vi "LIA7230Monitor.vi"(0 "Lock-in Reference":u16(ring) items=["Lock-in 1", "Lock-in 2", "Lock-in 3"]) -> ()   [LabVIEW 2019]
uses:
  Utility/Monitor Communication/LIA7230/LIA7230-cluster.ctl
  Utility/Monitor Communication/LIA7230/Settings_cluster.ctl
  Instrument_Setup.vi
  Global/Global Variables/Data_Display_global.vi
panel:
  out "LIA7230-Settings":T1={"Interface"=1, "Port"=0, "Serial Number"="08199244", "IP Address"="192.168.11.6", "Line Frequency\nRejection Filter"=0, "Input Mode"=1, "Input Conn. Shells"=TRUE, "Line Frequency"=FALSE, "Auto AC Gain"=FALSE, "AC Gain"=0, "Input Device"=FALSE, "Range"=26, " Auto Sensitivity "=FALSE, "Auto Measure"=FALSE, "Range 2"=25, " Auto Sensitivity  2"=FALSE, "Slope"=1, "Synchronous TC"=FALSE, "Time Constant"=12, "Slope 2"=1, "Time Constant 2"=12, "Oscillator Amp (V rms)"=0.5, "Oscillator Freq (Hz)"=150000.0, "Reference I/P"=0, "Ref Harm 1"=1, "Ref Harm2"=2, "Virtual Ref.\nMode"=FALSE, "Dual Harmonic/Reference Mode"=FALSE, "Reference Mode"=FALSE, "TRIG OUT\n= Ref Mon"=FALSE, " Auto Phase "=FALSE, "Reference Phase 1"=0.0, "+90 degrees 1"=FALSE, " Auto Phase 2 "=FALSE, "Reference 2 Phase"=0.0, "+90 degrees2"=FALSE, "Auxiliary I/O"=FALSE, "Configuration"=FALSE, "Curve Buffer"=FALSE, "Offsets"=FALSE, "X Channel Offset (%)"=-6.7055225e-06, "X Channel Offset"=FALSE, "Y Channel Offset (%)"=-6.705522537231445e-06, "Y Channel Offset"=FALSE, " Auto Offset"=FALSE, "X Channel Offset (%) 2"=-6.7055225e-06, "X Channel Offset 2"=FALSE, "Y Channel Offset (%) 2"=-6.705522537231445e-06, "Y Channel Offset 2"=FALSE, " Auto Offset 2"=FALSE, "Display Type channel 1"=5, "Display Type channel 2"=5, "Display Type channel 3"=5, "Display Type channel 4"=5, "Osc Sweeps"=FALSE, "Define Equation1"=FALSE, "Coupling"=FALSE} {"Display Type channel 4" items=["X %", "Y %", "X Calibrated", "Y Calibrated", "Mag %", "Mag Calibrated", "Phase Degrees", "Ratio", "Log Ratio", "ADC 1", "ADC 2", "ADC 3", "ADC 4", "Noise %", "Noise Calibrated", "Ref Frequency", "Equation 1", "Equation 2", "X2 %", "Y2 %", "X2 Calibrated", "Y2 Calibrated", "Mag2 %", "Mag2 Calibrated", "Phase2 Degrees"]; "Display Type channel 3" items=["X %", "Y %", "X Calibrated", "Y Calibrated", "Mag %", "Mag Calibrated", "Phase Degrees", "Ratio", "Log Ratio", "ADC 1", "ADC 2", "ADC 3", "ADC 4", "Noise %", "Noise Calibrated", "Ref Frequency", "Equation 1", "Equation 2", "X2 %", "Y2 %", "X2 Calibrated", "Y2 Calibrated", "Mag2 %", "Mag2 Calibrated", "Phase2 Degrees"]; "Display Type channel 2" items=["X %", "Y %", "X Calibrated", "Y Calibrated", "Mag %", "Mag Calibrated", "Phase Degrees", "Ratio", "Log Ratio", "ADC 1", "ADC 2", "ADC 3", "ADC 4", "Noise %", "Noise Calibrated", "Ref Frequency", "Equation 1", "Equation 2", "X2 %", "Y2 %", "Mag2 %", "Mag2 Calibrated", "Phase2 Degrees"]; "Display Type channel 1" items=["X %", "Y %", "X Calibrated", "Y Calibrated", "Mag %", "Mag Calibrated", "Phase Degrees", "Ratio", "Log Ratio", "ADC 1", "ADC 2", "ADC 3", "ADC 4", "Noise %", "Noise Calibrated", "Ref Frequency", "Equation 1", "Equation 2", "X2 %", "Y2 %", "Mag2 %", "Mag2 Calibrated", "Phase2 Degrees"]; "Y Channel Offset (%) 2" format="%.2f"; "X Channel Offset (%) 2" min=-300 max=300 step=0.01 format="%.2f"; "Y Channel Offset (%)" format="%.2f"; "X Channel Offset (%)" min=-300 max=300 step=0.01 format="%.2f"; "Reference 2 Phase" min=-200.0 max=200.0 step=0.01 scale=-180.0..180.0 scale format="%.1f"; "Reference Phase 1" min=-200.0 max=200.0 step=0.01 scale=-180.0..180.0 scale format="%.1f"; "Ref Harm2" min=1 max=127 step=1; "Ref Harm 1" min=1 max=127 step=1; "Reference I/P" items=["Internal", "External TTL (Rear Panel)", "External (Front Panel)"]; "Oscillator Freq (Hz)" min=0.5 max=150000.0 step=0.001 format="%.3f"; "Oscillator Amp (V rms)" min=0.0 max=5.0 step=0.0001 format="%.3f"; "Time Constant 2" items=["10µs", "20µs", "50µs", "100µs", "200µs", "500µs", "1ms", "2ms", "5ms", "10ms", "20ms", "50ms", "100ms", "200ms", "500ms", "1s", "2s", "5s", "10s", "20s", "50s", "100s", "200s", "500s", "1ks", "2ks", "5ks", "10ks", "20ks", "50ks", "100ks"]; "Slope 2" items=["6db/octave", "12dB/octave", "18dB/octave", "24dB/octave"]; "Time Constant" items=["10µs", "20µs", "50µs", "100µs", "200µs", "500µs", "1ms", "2ms", "5ms", "10ms", "20ms", "50ms", "100ms", "200ms", "500ms", "1s", "2s", "5s", "10s", "20s", "50s", "100s", "200s", "500s", "1ks", "2ks", "5ks", "10ks", "20ks", "50ks", "100ks"]; "Slope" items=["6db/octave", "12dB/octave", "18dB/octave", "24dB/octave"]; "Range 2" items=["N/A", "2nV", "5nV", "10nV", "20nV", "50nV", "100nV", "200nV", "500nV", "1µV", "2µV", "5µV", "10µV", "20µV", "50µV", "100µV", "200µV", "500µV", "1mV", "2mV", "5mV", "10mV", "20mV", "50mV", "100mV", "200mV", "500mV", "1V"]; "Range" items=["N/A", "2nV", "5nV", "10nV", "20nV", "50nV", "100nV", "200nV", "500nV", "1µV", "2µV", "5µV", "10µV", "20µV", "50µV", "100µV", "200µV", "500µV", "1mV", "2mV", "5mV", "10mV", "20mV", "50mV", "100mV", "200mV", "500mV", "1V"]; "AC Gain" items=["0dB", "6dB", "12dB", "18dB", "24dB", "30dB", "36dB", "42dB", "48dB", "54dB", "60dB", "66dB", "78dB", "84dB", "90dB"]; "Input Mode" items=["Inputs Grounded (test)", "A (Single-Ended Voltage)", "-B (Inverting Single Ended Voltage)", "A-B (Differential Voltage)", "AUX Input - Main Console", "B Current input - Wide Bandwidth", "B Current input - Low Noise"]; "Line Frequency\nRejection Filter" items=["OFF", "F", "2F", "F & 2F"]; "Port" items=["COM 1", "COM 2", "COM 3", "COM 4", "COM 5", "COM 6", "COM 7", "COM 8", "COM 9", "COM 10"]; "Interface" items=["RS232", "USB", "Ethernet"]}
  out "Sensitivity Range dual mode":i16(ring)=15 items=["2 nV", "5 nV", "10 nV", "20 nV", "50 nV", "100 nV", "200 nV", "500 nV", "1 µV", "2 µV", "5 µV", "10 µV", "20 µV", "50 µV", "100 µV", "200 µV", "500 µV", "1 mV", "2 mV", "5 mV", "10 mV", "20 mV", "50 mV", "100 mV", "200 mV", "500 mV", "1 V", ""]
  out "LIA7230-Cluser":T2={"Lockin 1"=[], "X1-Display"=0.0, "X1 Percent"=0.0, "Y1-Display"=0.0, "X1 Percent 2"=0.0, "Unit X1"="nV", "Unit X2"="nV", "X1 Overload"=FALSE, "Y1 Overload"=FALSE, "Sensitivity Setpoint"=26, "X1"=0.0, "Y1"=0.0, "Channel 3"=0.0, "Channel 4"=0.0, "Channel 4 Percent"=0.0, "Channel 3 Percent "=0.0, "Unit Channel 3"="nV", "Unit Channel 4"="nV", "Overload channel 3"=FALSE, "Overload channel 4"=FALSE, "Offsets (ON)"=FALSE, "Sensitivity Setpoint 2"=26} {"Sensitivity Setpoint 2" items=["2 nV", "5 nV", "10 nV", "20 nV", "50 nV", "100 nV", "200 nV", "500 nV", "1 µV", "2 µV", "5 µV", "10 µV", "20 µV", "50 µV", "100 µV", "200 µV", "500 µV", "1 mV", "2 mV", "5 mV", "10 mV", "20 mV", "50 mV", "100 mV", "200 mV", "500 mV", "1 V", ""]; "Channel 3 Percent" scale=0.0..100.0; "Channel 4 Percent" scale=0.0..100.0; "Sensitivity Setpoint" items=["2 nV", "5 nV", "10 nV", "20 nV", "50 nV", "100 nV", "200 nV", "500 nV", "1 µV", "2 µV", "5 µV", "10 µV", "20 µV", "50 µV", "100 µV", "200 µV", "500 µV", "1 mV", "2 mV", "5 mV", "10 mV", "20 mV", "50 mV", "100 mV", "200 mV", "500 mV", "1 V", ""]; "X1 Percent 2" scale=0.0..100.0; "X1 Percent" scale=0.0..100.0; "X1-Display" format="%#4_5f"}
  out "Sensitivity Range single mode":i16(ring)=15 items=["2 nV", "5 nV", "10 nV", "20 nV", "50 nV", "100 nV", "200 nV", "500 nV", "1 µV", "2 µV", "5 µV", "10 µV", "20 µV", "50 µV", "100 µV", "200 µV", "500 µV", "1 mV", "2 mV", "5 mV", "10 mV", "20 mV", "50 mV", "100 mV", "200 mV", "500 mV", "1 V", ""]
  in  "Stopp":bool
  # "USB Interface"
  # "Ethernet Interface"
  # "Oscillator"
  # "Output Channels -Offset"
  # "Reference Control"
  # "Dual Reference/\nDual Harmonic"
  # "Single Reference/\nSingle Harmonic"
  # "Dual"
  # "Input Configuration"
  # "Output Channels TC & Slope"
  # "Single"
  # "On"
  # "On"
  # "Single mode"
  # "Dual mode"
  # "Off"
  # "Off"
  # "DC"
  # "Dual Ref. Mode"
  # "AC"
  # "Dual Harm. Mode"
  # "On"
  # "On"
  # "Off"
  # "Off"
  # "On"
  # "Float"
  # "On"
  # "On"
  # "Off"
  # "Ground"
  # "Off"
  # "Off"
  # "FET"
  # "Sensitivity"
  # "50 Hz"
  # "On"
  # "Dual mode"
  # "Single mode"
  # "Bipolar"
  # "60 Hz"
  # "Off"
  # "Degrees"
  # "Degrees"
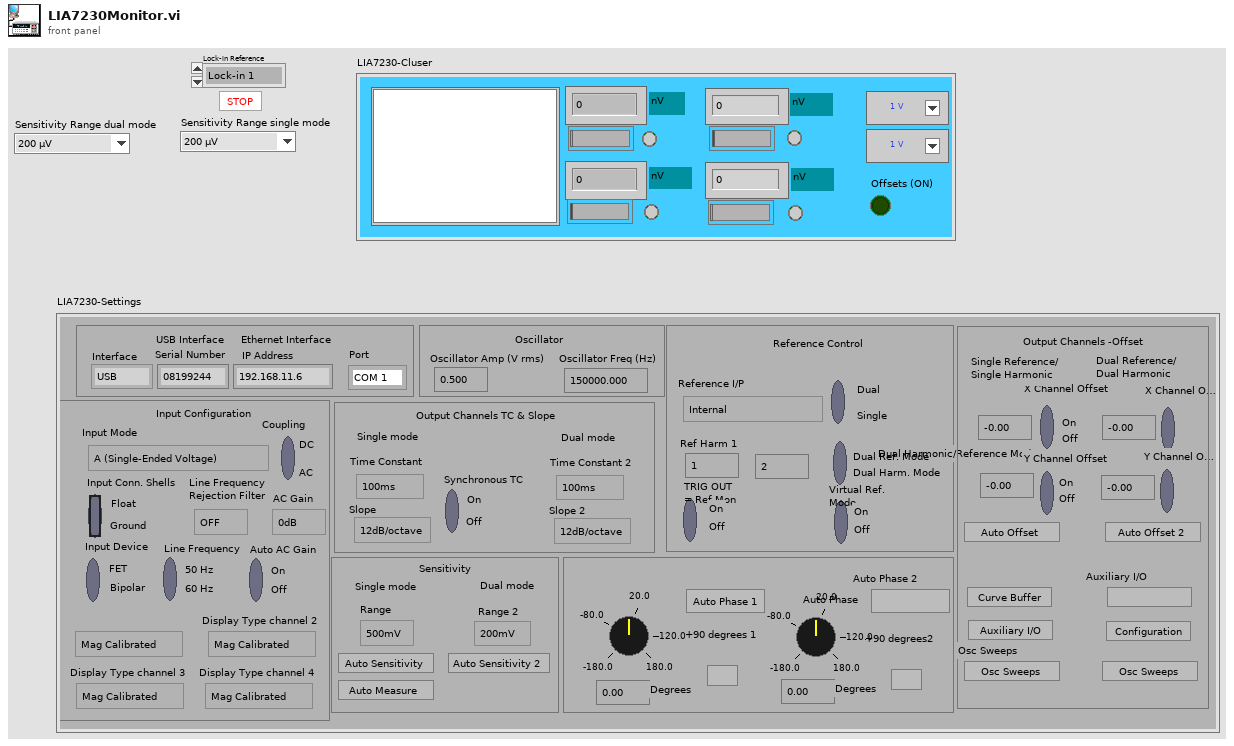
[diagram p1: front panel]
types:
  T1 = typedef "Settings_cluster.ctl" = cluster{"Interface":u16, "Port":u16, "Serial Number":string, "IP Address":string, "Line Frequency\nRejection Filter":u8, "Input Mode":u16, "Input Conn. Shells":bool, "Line Frequency":bool, "Auto AC Gain":bool, "AC Gain":u16, "Input Device":bool, "Range":u8, " Auto Sensitivity ":bool, "Auto Measure":bool, "Range 2":u8, " Auto Sensitivity  2":bool, "Slope":u8, "Synchronous TC":bool, "Time Constant":u16, "Slope 2":u8, "Time Constant 2":u16, "Oscillator Amp (V rms)":dbl, "Oscillator Freq (Hz)":dbl, "Reference I/P":u8, "Ref Harm 1":u16, "Ref Harm2":u16, "Virtual Ref.\nMode":bool, "Dual Harmonic/Reference Mode":bool, "Reference Mode":bool, "TRIG OUT\n= Ref Mon":bool, " Auto Phase ":bool, "Reference Phase 1":dbl, "+90 degrees 1":bool, " Auto Phase 2 ":bool, "Reference 2 Phase":dbl, "+90 degrees2":bool, "Auxiliary I/O":bool, "Configuration":bool, "Curve Buffer":bool, "Offsets":bool, "X Channel Offset (%)":sgl, "X Channel Offset":bool, "Y Channel Offset (%)":dbl, "Y Channel Offset":bool, " Auto Offset":bool, "X Channel Offset (%) 2":sgl, "X Channel Offset 2":bool, "Y Channel Offset (%) 2":dbl, "Y Channel Offset 2":bool, " Auto Offset 2":bool, "Display Type channel 1":u16, "Display Type channel 2":u16, "Display Type channel 3":u16, "Display Type channel 4":u16, "Osc Sweeps":bool, "Define Equation1":bool, "Coupling":bool}
  T2 = typedef "LIA7230-cluster.ctl" = cluster{"Lockin 1":dbl[][], "X1-Display":dbl, "X1 Percent":dbl, "Y1-Display":dbl, "X1 Percent 2":dbl, "Unit X1":string, "Unit X2":string, "X1 Overload":bool, "Y1 Overload":bool, "Sensitivity Setpoint":i16, "X1":dbl, "Y1":dbl, "Channel 3":dbl, "Channel 4":dbl, "Channel 4 Percent":dbl, "Channel 3 Percent ":dbl, "Unit Channel 3":string, "Unit Channel 4":string, "Overload channel 3":bool, "Overload channel 4":bool, "Offsets (ON)":bool, "Sensitivity Setpoint 2":i16}
  T3 = cluster{"Interface":u16, "Port":u16, "Serial Number":string, "IP Address":string, "Line Frequency\nRejection Filter":u8, "Input Mode":u16, "Input Conn. Shells":bool, "Line Frequency":bool, "Auto AC Gain":bool, "AC Gain":u16, "Input Device":bool, "Range":u8, " Auto Sensitivity ":bool, "Auto Measure":bool, "Range 2":u8, " Auto Sensitivity  2":bool, "Slope":u8, "Synchronous TC":bool, "Time Constant":u16, "Slope 2":u8, "Time Constant 2":u16, "Oscillator Amp (V rms)":dbl, "Oscillator Freq (Hz)":dbl, "Reference I/P":u8, "Ref Harm 1":u16, "Ref Harm2":u16, "Virtual Ref.\nMode":bool, "Dual Harmonic/Reference Mode":bool, "Reference Mode":bool, "TRIG OUT\n= Ref Mon":bool, " Auto Phase ":bool, "Reference Phase 1":dbl, "+90 degrees 1":bool, " Auto Phase 2 ":bool, "Reference 2 Phase":dbl, "+90 degrees2":bool, "Auxiliary I/O":bool, "Configuration":bool, "Curve Buffer":bool, "Offsets":bool, "X Channel Offset (%)":sgl, "X Channel Offset":bool, "Y Channel Offset (%)":dbl, "Y Channel Offset":bool, " Auto Offset":bool, "X Channel Offset (%) 2":sgl, "X Channel Offset 2":bool, "Y Channel Offset (%) 2":dbl, "Y Channel Offset 2":bool, " Auto Offset 2":bool, "Display Type channel 1":u16, "Display Type channel 2":u16, "Display Type channel 3":u16, "Display Type channel 4":u16, "Osc Sweeps":bool, "Define Equation1":bool, "Coupling":bool}
  T4 = cluster{"Sensitivity Setpoint 1":i32, "Sensitivity Setpoint 2":i32, "Sensitivity Setpoint 3":i32}
  T5 = cluster{"LIA7230-Running":bool, "LIA7230-Running 2":bool, "LIA7230-Running 3":bool, "SR830-Running":bool, "SR830-Running 2":bool, "SR830-Running 3":bool, "PE7265-running":bool, "zurich_Lock_in-running":bool}
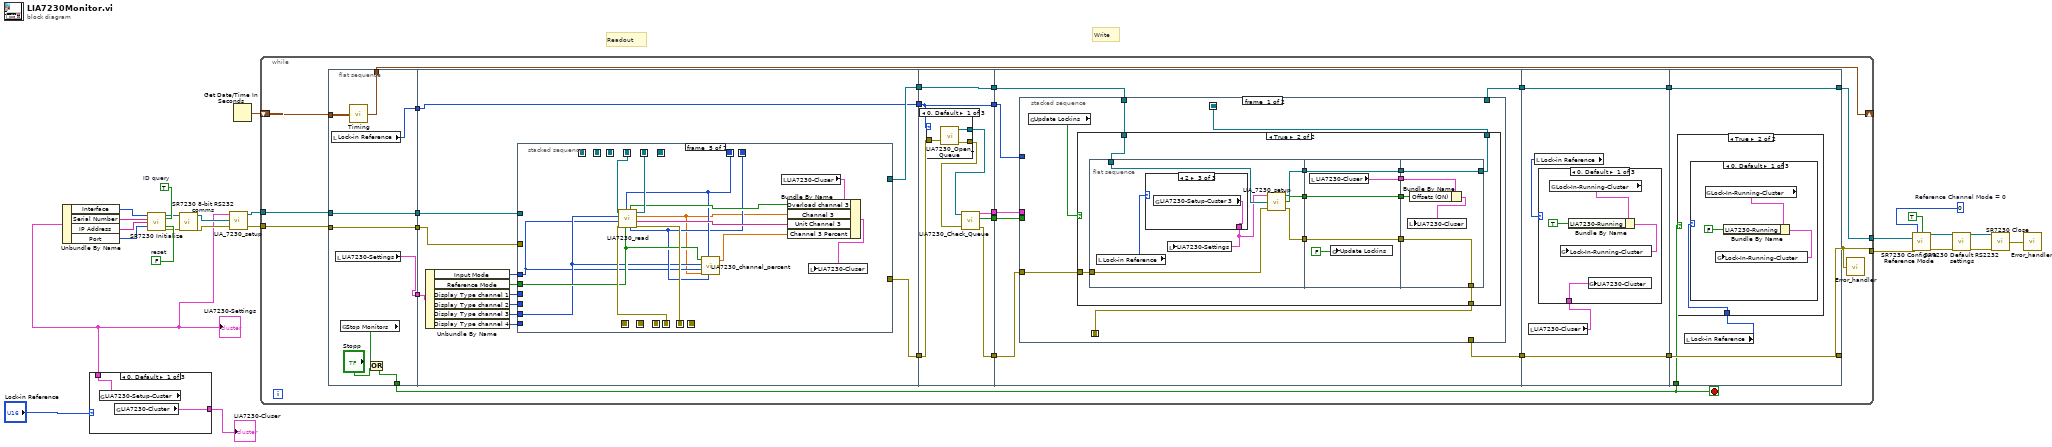
[diagram p0: block diagram]
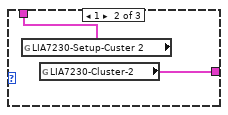
[diagram p2: hidden frame]
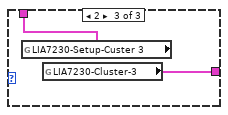
[diagram p3: hidden frame]
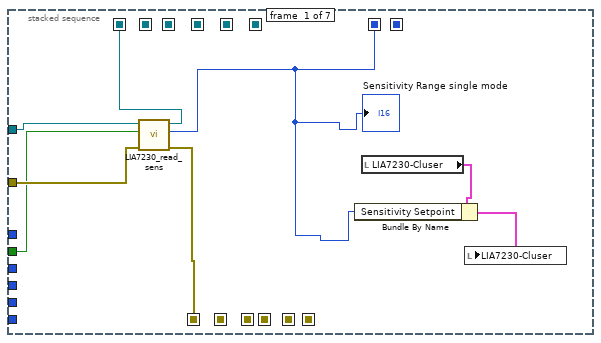
[diagram p4: hidden frame]
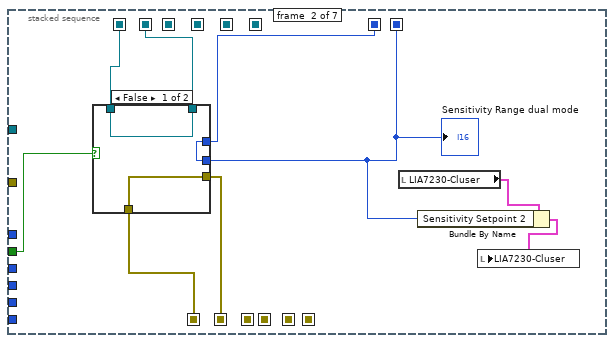
[diagram p5: hidden frame]
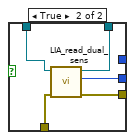
[diagram p6: hidden frame]
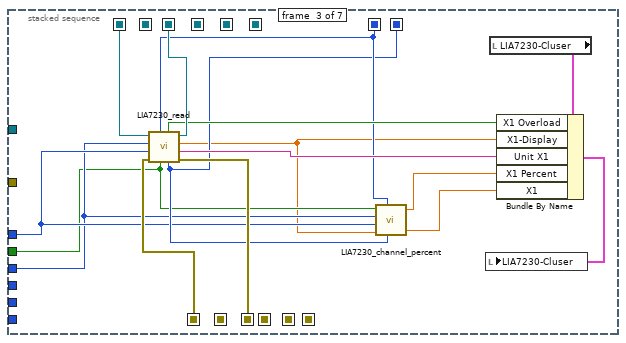
[diagram p7: hidden frame]
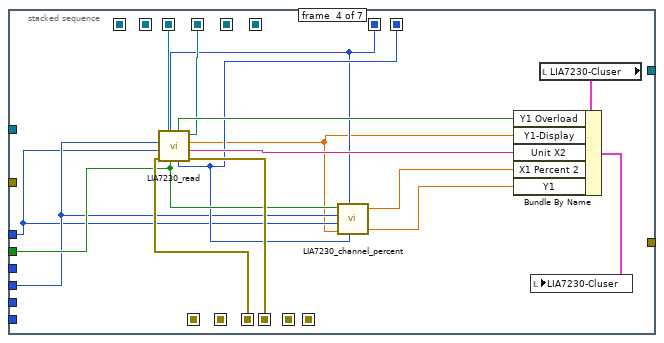
[diagram p8: hidden frame]
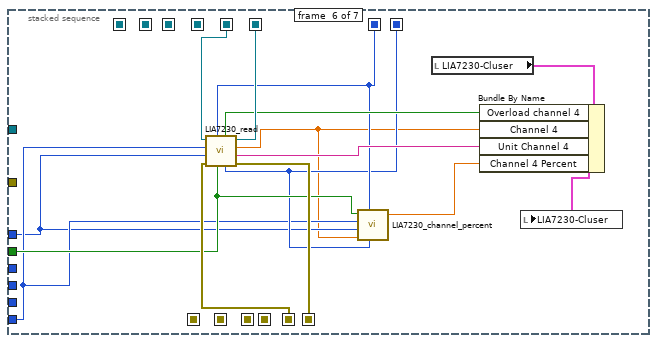
[diagram p9: hidden frame]
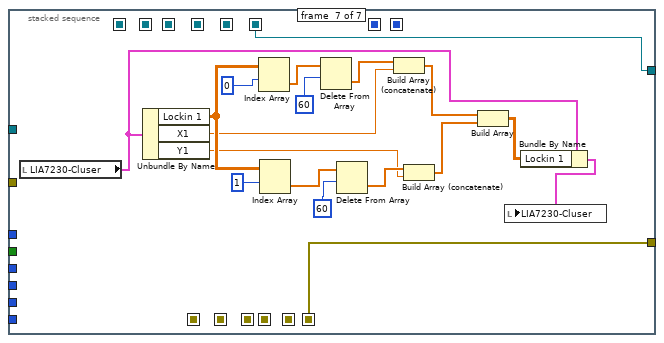
[diagram p10: hidden frame]
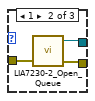
[diagram p11: hidden frame]
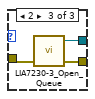
[diagram p12: hidden frame]
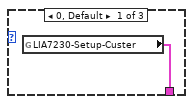
[diagram p14: hidden frame]
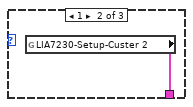
[diagram p15: hidden frame]
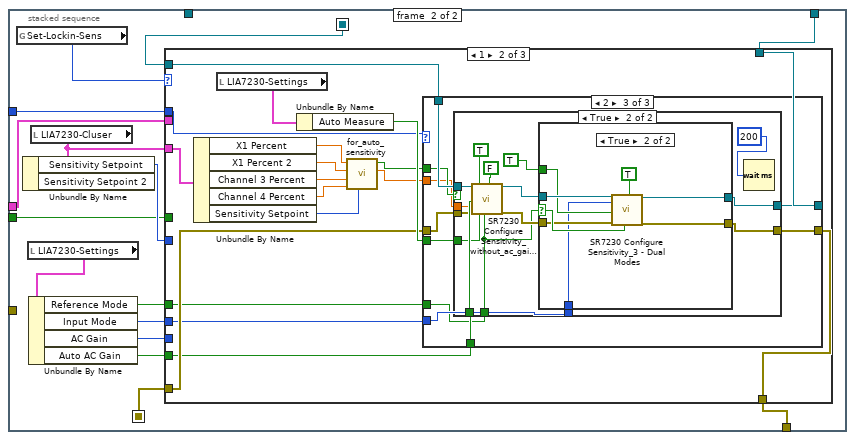
[diagram p16: hidden frame]
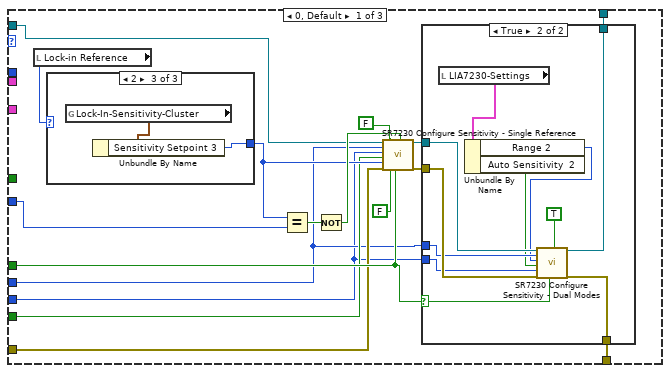
[diagram p17: hidden frame]
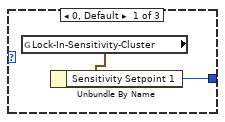
[diagram p19: hidden frame]
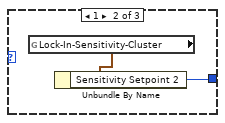
[diagram p20: hidden frame]
diagram:
  w14 = u16 0  # Reference Channel Mode = 0
  w18 = FALSE  # reset
  w19 = TRUE  # ID query
  # "Write"
  # "Readout"
  n1 = case shown="0, Default" "Lock-in Reference" {
    tunnel: [w27 w28 w31] -> w1
    tunnel: [w26 w29 w30] -> w17
    frame 0, Default {
      n2 = global read "Instrument_Setup.vi" "LIA7230-Setup-Custer"() -> (w27:T3)
      n3 = global read "Data_Display_global.vi" "LIA7230-Cluster"() -> (w26:T2)
    }
    frame 1 {
      n4 = global read "Instrument_Setup.vi" "LIA7230-Setup-Custer 2"() -> (w28:T3)
      n5 = global read "Data_Display_global.vi" "LIA7230-Cluster-2"() -> (w29:T2)
    }
    frame 2 {
      n6 = global read "Instrument_Setup.vi" "LIA7230-Setup-Custer 3"() -> (w31:T3)
      n7 = global read "Data_Display_global.vi" "LIA7230-Cluster-3"() -> (w30:T2)
    }
  }
  "LIA7230-Cluser" <- w17
  "LIA7230-Settings" <- w1
  n8 = Unbundle By Name(w1) -> ("Interface"=w23:u16, "Serial Number"=w22:string, "IP Address"=w21:string, "Port"=w20:u16)
  n9 = call "SR7230 Initialize.vi"("Interface"=w23, "Serial Number"=w22, "ID query"=w19, "IP Address"=w21, "Port"=w20, "reset"=w18) -> ("VISA session"=w16:refnum<visa-resource-name>, "error out"=w15:errorcluster)  [unwired: 7 in, 1 out]
  n10 = call "SR7230 8-bit RS232 comms.vi"("VISA session (for class)"=w16, "error in (no error)"=w15) -> ("VISA session"=w5:refnum<visa-resource-name>, "error out"=w2:errorcluster)  [unwired: 16 in]
  n11 = call "LIA_7230_setup.vi"("error in (no error)"=w2, "VISA  session"=w5, "LIA7230-Settings"=w1) -> ("error out"=w3:errorcluster, "Visa session (out)"=w4:refnum<visa-resource-name>)  [unwired: 1 out]
  n12 = Get Date/Time In Seconds() -> (seconds since 1Jan1904=w24:timestamp)
  n13 = while {
    shift-right: [w45] -> _
    shift-left: w24 -> [w54]
    tunnel: w4 -> [w52]
    tunnel: w3 -> [w50]
    tunnel: [w43] -> w13
    tunnel: [w42] -> w12
    stop <- w37 stop-if-true
    n14 = flat-sequence {
      tunnel: [w58] -> w37
      tunnel: w54 -> [w63]
      tunnel: [w62] -> w45
      tunnel: [w61] -> w53
      tunnel: w52 -> [w61]
      tunnel: [w60] -> w51
      tunnel: w50 -> [w60]
      tunnel: [w56] -> w44
      tunnel: [w55] -> w36
      tunnel: w53 -> [w75]
      tunnel: w51 -> [w74]
      tunnel: [w73] -> w49
      tunnel: [w72] -> w48
      tunnel: w44 -> [w71]
      tunnel: w36 -> [w64]
      tunnel: [w64] -> w35
      tunnel: w49 -> [w188]
      tunnel: w48 -> [w187]
      tunnel: [w188] -> w47
      tunnel: [w183] -> w46
      tunnel: w35 -> [w181]
      tunnel: [w186] -> w34
      tunnel: [w182] -> w33
      tunnel: [w181] -> w32
      tunnel: w47 -> [w204]
      tunnel: w46 -> [w202]
      tunnel: [w203] -> w41
      tunnel: [w201] -> w40
      tunnel: w34 -> [w200]
      tunnel: w33 -> [w199]
      tunnel: w32 -> [w198]
      tunnel: w41 -> [w467]
      tunnel: w40 -> [w466]
      tunnel: [w467] -> w39
      tunnel: [w466] -> w38
      tunnel: [w482] -> w42
      tunnel: [w483] -> w43
      tunnel: w39 -> [w483]
      tunnel: w38 -> [w482]
      tunnel: w37 -> [w481]
      frame #0 {
        n15 = local read "Lock-in Reference"() -> (w55:u16)
        n16 = local read "LIA7230-Settings"() -> (w56:T1)
        n17 = global read "Data_Display_global.vi" "Stop Monitors"() -> (w59:bool)
        n18 = call "Timing.vi"("start time (s)"=w63) -> ("last reading (s)"=w62:timestamp)
        n19 = Or(x=w59, y="Stopp") -> (x .or. y?=w58:bool)
      }
      frame #1 {
        n20 = Unbundle By Name(w71) -> ("Input Mode"=w70:u16, "Reference Mode"=w69:bool, "Display Type channel 1"=w68:u16, "Display Type channel 2"=w67:u16, "Display Type channel 3"=w66:u16, "Display Type channel 4"=w65:u16)
        n21 = stacked-sequence {
          seq-local: [w82 _ _ _ _ _ _] -> [_ w91 w116 _ _ _ _]
          seq-local: [_ _ w114 _ _ _ _] -> [_ _ _ w132 _ _ _]
          seq-local: [w80 _ _ _ _ _ _] -> [_ w90 w115 _ _ _ _]
          seq-local: [w76 _ _ _ _ _ _] -> [_ w87 w108 w122 w139 w153 _]
          seq-local: [_ _ w110 _ _ _ _] -> [_ _ _ w131 _ _ _]
          seq-local: [_ _ _ w126 _ _ _] -> [_ _ _ _ w145 _ _]
          seq-local: [_ _ _ w125 _ _ _] -> [_ _ _ _ w147 _ _]
          seq-local: [_ w88 _ _ _ _ _] -> [_ _ _ _ _ _ _]
          seq-local: [_ w89 _ _ _ _ _] -> [_ _ _ _ _ _ _]
          seq-local: [_ w85 _ _ _ _ _] -> [_ _ w107 w123 w138 w152 _]
          seq-local: [_ _ _ _ w146 _ _] -> [_ _ _ _ _ w160 _]
          seq-local: [_ _ _ _ w144 _ _] -> [_ _ _ _ _ w158 _]
          seq-local: [_ _ _ _ _ w159 _] -> [_ _ _ _ _ _ w164]
          seq-local: [_ _ _ _ _ w157 _] -> [_ _ _ _ _ _ w163]
          tunnel: w75 -> [w83 _ _ _ _ _ _]
          tunnel: w74 -> [w81 _ _ _ _ _ _]
          tunnel: w70 -> [_ _ w106 w120 w136 w150 _]
          tunnel: w69 -> [w77 w92 w104 w124 w140 w154 _]
          tunnel: [_ _ _ _ _ _ w164] -> w73
          tunnel: [_ _ _ _ _ _ w163] -> w72
          tunnel: w68 -> [_ _ w105 _ _ _ _]
          tunnel: w67 -> [_ _ _ w121 _ _ _]
          tunnel: w66 -> [_ _ _ _ w137 _ _]
          tunnel: w65 -> [_ _ _ _ _ w151 _]
          frame #0 {
            n22 = call "LIA7230_read_sens.vi"("error in (no error)"=w81, "Reference Mode"=w77, "VISA session (in)"=w83) -> ("error out"=w80:errorcluster, "Range Out"=w76:u8, "VISA session (out)"=w82:refnum<visa-resource-name>)  [unwired: 6 in]
            "Sensitivity Range single mode" <- w76
            n23 = local read "LIA7230-Cluser"() -> (w79:T2)
            n24 = Bundle By Name(cluster=w79, "Sensitivity Setpoint"=w76) -> (w78:T2)
            n25 = local write "LIA7230-Cluser"(w78) -> ()
          }
          frame #1 {
            n26 = case shown="False" w92 {
              tunnel: w91 -> [w94 w100]
              tunnel: w90 -> [w95 w99]
              tunnel: [w95 w98] -> w89
              tunnel: [w93 w97] -> w85
              tunnel: [w94 w96] -> w88
              tunnel: w87 -> [w93 _]
              frame False {
              }
              frame True {
                n27 = call "LIA_read_dual_sens.vi"("error in (no error)"=w99, "VISA session (in)"=w100) -> ("error out"=w98:errorcluster, "Range dual mode Out"=w97:u8, "VISA session (out)"=w96:refnum<visa-resource-name>)  [unwired: 7 in]
              }
            }
            "Sensitivity Range dual mode" <- w85
            n28 = local read "LIA7230-Cluser"() -> (w86:T2)
            n29 = Bundle By Name(cluster=w86, "Sensitivity Setpoint 2"=w85) -> (w84:T2)
            n30 = local write "LIA7230-Cluser"(w84) -> ()
          }
          frame #2 {
            n31 = call "LIA7230_read.vi"("Range dual mode"=w107, "Reference Mode"=w104, "Range single mode"=w108, "error in (no error)"=w115, "Input Mode"=w106, "Display Type"=w105, "VISA session (for class)"=w116) -> ("error out"=w110:errorcluster, "Units"=w111:string, "Display"=w103:dbl, "VISA session (out)"=w114:refnum<visa-resource-name>, "Overload"=w109:bool)
            n32 = call "LIA7230_channel_percent.vi"("Reference Mode"=w104, "Range single mode"=w108, "Display Type"=w105, "Input Mode"=w106, "Range dual mode"=w107, "Channel signal"=w103) -> ("Channel signal percent"=w102:dbl, "Channel signal in full range"=w101:dbl)  [unwired: 1 in]
            n33 = local read "LIA7230-Cluser"() -> (w113:T2)
            n34 = Bundle By Name(cluster=w113, "X1 Overload"=w109, "X1-Display"=w103, "Unit X1"=w111, "X1 Percent"=w102, "X1"=w101) -> (w112:T2)
            n35 = local write "LIA7230-Cluser"(w112) -> ()
          }
          frame #3 {
            n36 = call "LIA7230_read.vi"("Range dual mode"=w123, "Reference Mode"=w124, "Range single mode"=w122, "error in (no error)"=w131, "Input Mode"=w120, "Display Type"=w121, "VISA session (for class)"=w132) -> ("error out"=w126:errorcluster, "Units"=w127:string, "Display"=w119:dbl, "VISA session (out)"=w125:refnum<visa-resource-name>, "Overload"=w128:bool)
            n37 = call "LIA7230_channel_percent.vi"("Reference Mode"=w124, "Range single mode"=w122, "Display Type"=w121, "Input Mode"=w120, "Range dual mode"=w123, "Channel signal"=w119) -> ("Channel signal percent"=w118:dbl, "Channel signal in full range"=w117:dbl)  [unwired: 1 in]
            n38 = local read "LIA7230-Cluser"() -> (w130:T2)
            n39 = Bundle By Name(cluster=w130, "Y1 Overload"=w128, "Y1-Display"=w119, "Unit X2"=w127, "X1 Percent 2"=w118, "Y1"=w117) -> (w129:T2)
            n40 = local write "LIA7230-Cluser"(w129) -> ()
          }
          frame #4 {
            n41 = call "LIA7230_read.vi"("Range dual mode"=w138, "Reference Mode"=w140, "Range single mode"=w139, "error in (no error)"=w145, "Input Mode"=w136, "Display Type"=w137, "VISA session (for class)"=w147) -> ("error out"=w144:errorcluster, "Units"=w142:string, "Display"=w135:dbl, "VISA session (out)"=w146:refnum<visa-resource-name>, "Overload"=w141:bool)
            n42 = call "LIA7230_channel_percent.vi"("Reference Mode"=w140, "Range single mode"=w139, "Display Type"=w137, "Input Mode"=w136, "Range dual mode"=w138, "Channel signal"=w135) -> ("Channel signal percent"=w134:dbl)  [unwired: 1 in, 1 out]
            n43 = local read "LIA7230-Cluser"() -> (w143:T2)
            n44 = Bundle By Name(cluster=w143, "Overload channel 3"=w141, "Channel 3"=w135, "Unit Channel 3"=w142, "Channel 3 Percent"=w134) -> (w133:T2)
            n45 = local write "LIA7230-Cluser"(w133) -> ()
          }
          frame #5 {
            n46 = call "LIA7230_read.vi"("Range dual mode"=w152, "Reference Mode"=w154, "Range single mode"=w153, "error in (no error)"=w158, "Input Mode"=w150, "Display Type"=w151, "VISA session (for class)"=w160) -> ("error out"=w157:errorcluster, "Units"=w156:string, "Display"=w149:dbl, "VISA session (out)"=w159:refnum<visa-resource-name>, "Overload"=w155:bool)
            n47 = call "LIA7230_channel_percent.vi"("Reference Mode"=w154, "Range single mode"=w153, "Display Type"=w151, "Input Mode"=w150, "Range dual mode"=w152, "Channel signal"=w149) -> ("Channel signal percent"=w148:dbl)  [unwired: 1 in, 1 out]
            n48 = local read "LIA7230-Cluser"() -> (w162:T2)
            n49 = Bundle By Name(cluster=w162, "Overload channel 4"=w155, "Channel 4"=w149, "Unit Channel 4"=w156, "Channel 4 Percent"=w148) -> (w161:T2)
            n50 = local write "LIA7230-Cluser"(w161) -> ()
          }
          frame #6 {
            n51 = local read "LIA7230-Cluser"() -> (w167:T2)
            n52 = Unbundle By Name(w167) -> ("Lockin 1"=w179:dbl[][], "X1"=w172:dbl, "Y1"=w170:dbl)
            n53 = Index Array(array=w179, index (row)=0) -> (element=w177:dbl[])  [unwired: 1 in]
            n54 = Index Array(array=w179, index (row)=1) -> (element=w175:dbl[])  [unwired: 1 in]
            n55 = Delete From Array(array=w177, length=60) -> (deleted portion=w173:dbl[])  [unwired: 1 in, 1 out]
            n56 = Delete From Array(array=w175, length=60) -> (deleted portion=w171:dbl[])  [unwired: 1 in, 1 out]
            n57 = Build Array (concatenate)(w173, w172) -> (w169:dbl[])
            n58 = Build Array (concatenate)(w171, w170) -> (w168:dbl[])
            n59 = Build Array(w169, w168) -> (w165:dbl[][])
            n60 = Bundle By Name(cluster=w167, "Lockin 1"=w165) -> (w166:T2)
            n61 = local write "LIA7230-Cluser"(w166) -> ()
          }
        }
      }
      frame #2 {
        n62 = case shown="0, Default" w181 {
          tunnel: w187 -> [w191 w193 w196]
          tunnel: [w190 w194 w197] -> w184
          tunnel: [w189 w192 w195] -> w185
          frame 0, Default {
            n63 = call "LIA7230_Open_Queue.vi"("error in (no error)"=w191) -> ("error out"=w190:errorcluster, "queue out"=w189:refnum<queue>)  [unwired: 3 in]
          }
          frame 1 {
            n64 = call "LIA7230-2_Open_Queue.vi"("error in (no error)"=w193) -> ("error out"=w194:errorcluster, "queue out"=w192:refnum<queue>)  [unwired: 3 in]
          }
          frame 2 {
            n65 = call "LIA7230-3_Open_Queue.vi"("error in (no error)"=w196) -> ("error out"=w197:errorcluster, "queue out"=w195:refnum<queue>)  [unwired: 3 in]
          }
        }
        n66 = call "LIA7230_Check_Queue.vi"("queue"=w185, "error in (no error)"=w184) -> ("LIA7230-Cluser"=w186:T2, "New Entries?"=w182:bool, "error out"=w183:errorcluster)  [unwired: 2 in]
      }
      frame #3 {
        n67 = stacked-sequence {
          seq-local: [w206 _] -> [_ w255]
          seq-local: [w205 _] -> [_ w254]
          tunnel: w204 -> [w208 _]
          tunnel: [_ w246] -> w203
          tunnel: w202 -> [w207 _]
          tunnel: [_ w245] -> w201
          tunnel: w200 -> [_ w248]
          tunnel: w199 -> [_ w247]
          tunnel: w198 -> [_ w244]
          frame #0 {
            n68 = global read "Instrument_Setup.vi" "Update Lockins"() -> (w209:bool)
            n69 = case shown="True" w209 {
              tunnel: w208 -> [w211 w222]
              tunnel: [w211 w216] -> w205
              tunnel: w207 -> [w210 w215]
              tunnel: [w210 w212] -> w206
              frame False {
              }
              frame True {
                n70 = flat-sequence {
                  tunnel: w222 -> [w228]
                  tunnel: [w226] -> w219
                  tunnel: [w225] -> w217
                  tunnel: w215 -> [w224]
                  tunnel: [w223] -> w213
                  tunnel: [w236] -> w221
                  tunnel: [w235] -> w220
                  tunnel: w219 -> [w235]
                  tunnel: [w234] -> w218
                  tunnel: w217 -> [w234]
                  tunnel: [w233] -> w214
                  tunnel: w213 -> [w233]
                  tunnel: w221 -> [w242]
                  tunnel: w220 -> [w240]
                  tunnel: [w239] -> w216
                  tunnel: w218 -> [w239]
                  tunnel: w214 -> [w238]
                  tunnel: [w238] -> w212
                  frame #0 {
                    n71 = local read "Lock-in Reference"() -> (w229:u16)
                    n72 = case shown="2" w229 {
                      tunnel: [w230 w231 w232] -> w227
                      frame 0, Default {
                        n73 = global read "Instrument_Setup.vi" "LIA7230-Setup-Custer"() -> (w230:T3)
                      }
                      frame 1 {
                        n74 = global read "Instrument_Setup.vi" "LIA7230-Setup-Custer 2"() -> (w231:T3)
                      }
                      frame 2 {
                        n75 = global read "Instrument_Setup.vi" "LIA7230-Setup-Custer 3"() -> (w232:T3)
                      }
                    }
                    n76 = local write "LIA7230-Settings"(w227) -> ()
                    n77 = call "LIA_7230_setup.vi"("error in (no error)"=w224, "VISA  session"=w228, "LIA7230-Settings"=w227) -> ("error out"=w223:errorcluster, "Offsets (ON)"=w226:bool, "Visa session (out)"=w225:refnum<visa-resource-name>)
                  }
                  frame #1 {
                    n78 = local read "LIA7230-Cluser"() -> (w236:T2)
                    n79 = global write "Instrument_Setup.vi" "Update Lockins"(FALSE) -> ()
                  }
                  frame #2 {
                    n80 = Bundle By Name(cluster=w242, "Offsets (ON)"=w240) -> (w241:T2)
                    n81 = local write "LIA7230-Cluser"(w241) -> ()
                  }
                }
              }
            }
          }
          frame #1 {
            n82 = global read "Instrument_Setup.vi" "Set-Lockin-Sens"() -> (w257:u16)
            n83 = local read "LIA7230-Settings"() -> (w253:T1)
            n84 = Unbundle By Name(w253) -> ("Reference Mode"=w252:bool, "Input Mode"=w251:u16, "AC Gain"=w250:u16, "Auto AC Gain"=w249:bool)
            n85 = local read "LIA7230-Cluser"() -> (w243:T2)
            n86 = Unbundle By Name(w243) -> ("Sensitivity Setpoint"=w256:i16)  [unwired: 1 out]
            n87 = case shown="1" w257 {
              tunnel: w256 -> [w270 _ _]
              tunnel: w255 -> [w266 w309 w429]
              tunnel: w254 -> [w264 w308 w427]
              tunnel: w252 -> [w273 w307 w430]
              tunnel: w251 -> [w259 w306 w425]
              tunnel: w250 -> [w258 _ w424]
              tunnel: w249 -> [w263 w305 w423]
              tunnel: [w261 w304 w426] -> w246
              tunnel: [w260 w303 w428] -> w245
              tunnel: w248 -> [_ _ w432]
              tunnel: w247 -> [_ _ w431]
              tunnel: w244 -> [_ w302 _]
              tunnel: w243 -> [_ w301 _]
              frame 0, Default {
                n88 = local read "Lock-in Reference"() -> (w274:u16)
                n89 = case shown="2" w274 {
                  tunnel: [w288 w290 w292] -> w267
                  frame 0, Default {
                    n90 = global read "Data_Display_global.vi" "Lock-In-Sensitivity-Cluster"() -> (w289:T4)
                    n91 = Unbundle By Name(w289) -> ("Sensitivity Setpoint 1"=w288:i32)
                  }
                  frame 1 {
                    n92 = global read "Data_Display_global.vi" "Lock-In-Sensitivity-Cluster"() -> (w291:T4)
                    n93 = Unbundle By Name(w291) -> ("Sensitivity Setpoint 2"=w290:i32)
                  }
                  frame 2 {
                    n94 = global read "Data_Display_global.vi" "Lock-In-Sensitivity-Cluster"() -> (w293:T4)
                    n95 = Unbundle By Name(w293) -> ("Sensitivity Setpoint 3"=w292:i32)
                  }
                }
                n96 = Equal?(x=w267, y=w270) -> (x = y?=w269:bool)
                n97 = Not(x=w269) -> (.not. x?=w268:bool)
                n98 = call "SR7230 Configure Sensitivity - Single Reference.vi"("VISA session (for class)"=w264, "Input Mode"=w259, "AC Gain"=w258, "Auto AC Gain"=w263, "Range"=w267, "error in (no error)"=w266, "Auto Sensitivity"=FALSE, "Auto Measure"=FALSE, "Reference Mode"=w273, "Update"=w268) -> ("VISA session"=w262:refnum<visa-resource-name>, "error out"=w265:errorcluster)  [unwired: 3 in, 5 out]
                n99 = case shown="True" w273 {
                  selector: w273 -> [_ w287]
                  tunnel: w265 -> [w275 w285]
                  tunnel: w262 -> [w276 w286]
                  tunnel: [w276 w284] -> w261
                  tunnel: [w275 w283] -> w260
                  tunnel: w259 -> [_ w281]
                  tunnel: w258 -> [_ w280]
                  frame False {
                  }
                  frame True {
                    n100 = local read "LIA7230-Settings"() -> (w282:T1)
                    n101 = Unbundle By Name(w282) -> ("Range 2"=w279:u8, "Auto Sensitivity  2"=w278:bool)
                    n102 = call "SR7230 Configure Sensitivity - Dual Modes.vi"("VISA session (for class)"=w286, "Input Mode"=w281, "Range 2"=w279, "Auto Sensitivity 2"=w278, "AC Gain In"=w280, "error in (no error)"=w285, "Reference Mode"=w287, "Update"=TRUE) -> ("dup VISA session"=w284:refnum<visa-resource-name>, "error out"=w283:errorcluster)  [unwired: 6 in, 4 out]
                  }
                }
              }
              frame 1 {
                n103 = Unbundle By Name(w301) -> ("X1 Percent"=w300:dbl, "X1 Percent 2"=w299:dbl, "Channel 3 Percent"=w298:dbl, "Channel 4 Percent"=w297:dbl, "Sensitivity Setpoint"=w296:i16)
                n104 = local read "LIA7230-Settings"() -> (w311:T1)
                n105 = Unbundle By Name(w311) -> ("Auto Measure"=w310:bool)
                n106 = call "for_auto_sensitivity.vi"("Sensutivity old"=w296, "Ch4 percent"=w297, "Ch3 percent"=w298, "Ch2 percent"=w299, "Ch1 percent"=w300) -> ("Sensitivity new"=w294:dbl, "Change sensitivity"=w295:bool)  [unwired: 5 in]
                n107 = case shown="2" w302 {
                  tunnel: w310 -> [w321 w353 w390]
                  tunnel: w309 -> [w320 w354 w389]
                  tunnel: w308 -> [w319 w351 w388]
                  tunnel: w307 -> [w318 w352 w391]
                  tunnel: w306 -> [w317 w356 w392]
                  tunnel: w305 -> [w316 w355 w393]
                  tunnel: [w315 w358 w395] -> w304
                  tunnel: [w314 w357 w394] -> w303
                  tunnel: w295 -> [w313 w349 w387]
                  tunnel: w294 -> [w312 w350 w386]
                  frame 0, Default {
                    n108 = case shown="True" w313 {
                      tunnel: w321 -> [_ w338]
                      tunnel: w320 -> [w322 w337]
                      tunnel: w319 -> [w323 w336]
                      tunnel: w318 -> [_ w335]
                      tunnel: w317 -> [_ w331]
                      tunnel: w316 -> [_ w330]
                      tunnel: [w323 w329] -> w315
                      tunnel: [w322 w328] -> w314
                      tunnel: w312 -> [_ w324]
                      frame False {
                      }
                      frame True {
                        n109 = call "SR7230 Configure Sensitivity_without_ac_gain - Single Reference.vi"("VISA session (for class)"=w336, "Input Mode"=w331, "Auto AC Gain"=w330, "Range"=w324, "error in (no error)"=w337, "Auto Sensitivity"=FALSE, "Auto Measure"=w338, "Reference Mode"=w335, "Update"=FALSE) -> ("VISA session"=w333:refnum<visa-resource-name>, "error out"=w334:errorcluster)  [unwired: 4 in, 5 out]
                        n110 = case shown="True" w335 {
                          selector: w335 -> [_ w348]
                          tunnel: w334 -> [w339 w347]
                          tunnel: [w339 w346] -> w328
                          tunnel: w333 -> [w340 w345]
                          tunnel: [w340 w344] -> w329
                          tunnel: TRUE -> [_ w343]
                          tunnel: w331 -> [_ w341]
                          frame False {
                          }
                          frame True {
                            n111 = call "SR7230 Configure Sensitivity - Dual Modes.vi"("VISA session (for class)"=w345, "Input Mode"=w341, "Auto Sensitivity 2"=w343, "error in (no error)"=w347, "Reference Mode"=w348, "Update"=TRUE) -> ("dup VISA session"=w344:refnum<visa-resource-name>, "error out"=w346:errorcluster)  [unwired: 8 in, 4 out]
                          }
                        }
                        n112 = Wait (ms)(milliseconds to wait=200) -> ()  [unwired: 1 out]
                      }
                    }
                  }
                  frame 1 {
                    n113 = case shown="True" w349 {
                      tunnel: [w360 w370] -> w358
                      tunnel: [w359 w369] -> w357
                      tunnel: w356 -> [_ w368]
                      tunnel: w355 -> [_ w367]
                      tunnel: w354 -> [w359 w366]
                      tunnel: w353 -> [_ w365]
                      tunnel: w352 -> [_ w364]
                      tunnel: w351 -> [w360 w363]
                      tunnel: w350 -> [_ w362]
                      frame False {
                      }
                      frame True {
                        n114 = call "SR7230 Configure Sensitivity_without_ac_gain_2 - Single Reference.vi"("VISA session (for class)"=w363, "Auto AC Gain"=w367, "Range"=w362, "error in (no error)"=w366, "Auto Sensitivity"=TRUE, "Auto Measure"=w365, "Reference Mode"=w364, "Update"=FALSE) -> ("VISA session"=w374:refnum<visa-resource-name>, "error out"=w375:errorcluster)  [unwired: 5 in, 5 out]
                        n115 = case shown="True" w364 {
                          selector: w364 -> [_ w385]
                          tunnel: w375 -> [w376 w384]
                          tunnel: [w376 w383] -> w369
                          tunnel: w374 -> [w377 w382]
                          tunnel: [w377 w381] -> w370
                          tunnel: TRUE -> [_ w380]
                          tunnel: w368 -> [_ w378]
                          frame False {
                          }
                          frame True {
                            n116 = call "SR7230 Configure Sensitivity_2 - Dual Modes.vi"("VISA session (for class)"=w382, "Input Mode"=w378, "Auto Sensitivity 2"=w380, "error in (no error)"=w384, "Reference Mode"=w385, "Update"=TRUE) -> ("dup VISA session"=w381:refnum<visa-resource-name>, "error out"=w383:errorcluster)  [unwired: 8 in, 4 out]
                          }
                        }
                        n117 = Wait (ms)(milliseconds to wait=200) -> ()  [unwired: 1 out]
                      }
                    }
                  }
                  frame 2 {
                    n118 = case shown="True" w387 {
                      tunnel: [w397 w407] -> w395
                      tunnel: [w396 w406] -> w394
                      tunnel: w393 -> [_ w405]
                      tunnel: w392 -> [_ w404]
                      tunnel: w391 -> [_ w403]
                      tunnel: w390 -> [_ w402]
                      tunnel: w389 -> [w396 w401]
                      tunnel: w388 -> [w397 w400]
                      tunnel: w386 -> [_ w399]
                      frame False {
                      }
                      frame True {
                        n119 = call "SR7230 Configure Sensitivity_without_ac_gain_3 - Single Reference.vi"("VISA session (for class)"=w400, "Auto AC Gain"=w405, "Range"=w399, "error in (no error)"=w401, "Auto Sensitivity"=TRUE, "Auto Measure"=w402, "Reference Mode"=w403, "Update"=FALSE) -> ("VISA session"=w411:refnum<visa-resource-name>, "error out"=w412:errorcluster)  [unwired: 5 in, 5 out]
                        n120 = case shown="True" w403 {
                          selector: w403 -> [_ w422]
                          tunnel: w412 -> [w413 w421]
                          tunnel: [w413 w420] -> w406
                          tunnel: w411 -> [w414 w419]
                          tunnel: [w414 w418] -> w407
                          tunnel: TRUE -> [_ w417]
                          tunnel: w404 -> [_ w415]
                          frame False {
                          }
                          frame True {
                            n121 = call "SR7230 Configure Sensitivity_3 - Dual Modes.vi"("VISA session (for class)"=w419, "Input Mode"=w415, "Auto Sensitivity 2"=w417, "error in (no error)"=w421, "Reference Mode"=w422, "Update"=TRUE) -> ("dup VISA session"=w418:refnum<visa-resource-name>, "error out"=w420:errorcluster)  [unwired: 8 in, 4 out]
                          }
                        }
                        n122 = Wait (ms)(milliseconds to wait=200) -> ()  [unwired: 1 out]
                      }
                    }
                  }
                }
              }
              frame 2 {
                n123 = case shown="True" w431 {
                  tunnel: w432 -> [_ w451]
                  tunnel: w430 -> [_ w450]
                  tunnel: w429 -> [w433 w449]
                  tunnel: [w433 w447] -> w428
                  tunnel: w427 -> [w434 w446]
                  tunnel: [w434 w444] -> w426
                  tunnel: w425 -> [_ w436]
                  tunnel: w424 -> [_ w440]
                  tunnel: w423 -> [_ w439]
                  frame False {
                  }
                  frame True {
                    n124 = Unbundle By Name(w451) -> ("Sensitivity Setpoint"=w438:i16, "Sensitivity Setpoint 2"=w435:i16)
                    n125 = call "SR7230 Configure Sensitivity - Single Reference.vi"("VISA session (for class)"=w446, "Input Mode"=w436, "AC Gain"=w440, "Auto AC Gain"=w439, "Range"=w438, "error in (no error)"=w449, "Auto Sensitivity"=FALSE, "Auto Measure"=FALSE, "Reference Mode"=w450, "Update"=TRUE) -> ("VISA session"=w445:refnum<visa-resource-name>, "ACGAIN out"=w437:i32, "error out"=w448:errorcluster)  [unwired: 3 in, 4 out]
                    n126 = case shown="True" w450 {
                      selector: w450 -> [_ w463]
                      tunnel: w448 -> [w452 w462]
                      tunnel: [w452 w461] -> w447
                      tunnel: w445 -> [w453 w460]
                      tunnel: [w453 w459] -> w444
                      tunnel: w437 -> [_ w457]
                      tunnel: w436 -> [_ w455]
                      tunnel: w435 -> [_ w454]
                      frame False {
                      }
                      frame True {
                        n127 = call "SR7230 Configure Sensitivity - Dual Modes.vi"("VISA session (for class)"=w460, "Input Mode"=w455, "Range 2"=w454, "Auto Sensitivity 2"=FALSE, "AC Gain In"=w457, "error in (no error)"=w462, "Reference Mode"=w463, "Update"=TRUE) -> ("dup VISA session"=w459:refnum<visa-resource-name>, "error out"=w461:errorcluster)  [unwired: 6 in, 4 out]
                      }
                    }
                  }
                }
              }
            }
          }
        }
      }
      frame #4 {
        n128 = local read "LIA7230-Cluser"() -> (w464:T2)
        n129 = local read "Lock-in Reference"() -> (w465:u16)
        n130 = case shown="0, Default" w465 {
          tunnel: w464 -> [w468 w472 w479]
          frame 0, Default {
            n131 = global read "Data_Display_global.vi" "Lock-In-Running-Cluster"() -> (w471:T5)
            n132 = Bundle By Name(cluster=w471, "LIA7230-Running"=TRUE) -> (w469:T5)
            n133 = global write "Data_Display_global.vi" "Lock-In-Running-Cluster"(w469) -> ()
            n134 = global write "Data_Display_global.vi" "LIA7230-Cluster"(w468) -> ()
          }
          frame 1 {
            n135 = global read "Data_Display_global.vi" "Lock-In-Running-Cluster"() -> (w475:T5)
            n136 = Bundle By Name(cluster=w475, "LIA7230-Running 2"=TRUE) -> (w473:T5)
            n137 = global write "Data_Display_global.vi" "Lock-In-Running-Cluster"(w473) -> ()
            n138 = global write "Data_Display_global.vi" "LIA7230-Cluster-2"(w472) -> ()
          }
          frame 2 {
            n139 = global read "Data_Display_global.vi" "Lock-In-Running-Cluster"() -> (w478:T5)
            n140 = Bundle By Name(cluster=w478, "LIA7230-Running 3"=TRUE) -> (w476:T5)
            n141 = global write "Data_Display_global.vi" "Lock-In-Running-Cluster"(w476) -> ()
            n142 = global write "Data_Display_global.vi" "LIA7230-Cluster-3"(w479) -> ()
          }
        }
      }
      frame #5 {
        n143 = local read "Lock-in Reference"() -> (w480:u16)
        n144 = case shown="True" w481 {
          tunnel: w480 -> [_ w484]
          frame False {
          }
          frame True {
            n145 = case shown="0, Default" w484 {
              frame 0, Default {
                n146 = global read "Data_Display_global.vi" "Lock-In-Running-Cluster"() -> (w487:T5)
                n147 = Bundle By Name(cluster=w487, "LIA7230-Running"=FALSE) -> (w485:T5)
                n148 = global write "Data_Display_global.vi" "Lock-In-Running-Cluster"(w485) -> ()
              }
              frame 1 {
                n149 = global read "Data_Display_global.vi" "Lock-In-Running-Cluster"() -> (w490:T5)
                n150 = Bundle By Name(cluster=w490, "LIA7230-Running 2"=FALSE) -> (w488:T5)
                n151 = global write "Data_Display_global.vi" "Lock-In-Running-Cluster"(w488) -> ()
              }
              frame 2 {
                n152 = global read "Data_Display_global.vi" "Lock-In-Running-Cluster"() -> (w493:T5)
                n153 = Bundle By Name(cluster=w493, "LIA7230-Running 3"=FALSE) -> (w491:T5)
                n154 = global write "Data_Display_global.vi" "Lock-In-Running-Cluster"(w491) -> ()
              }
            }
          }
        }
      }
    }
    n155 = call "Error_handler.vi"("error constant"=w42) -> ()
  }
  n156 = call "SR7230 Configure Reference Mode.vi"("VISA session (for class)"=w13, "Reference Channel Mode"=w14, "error in (no error)"=w12, "Update"=TRUE) -> ("dup VISA session"=w10:refnum<visa-resource-name>, "error out"=w9:errorcluster)  [unwired: 14 in]
  n157 = call "SR7230 Default RS2232 settings.vi"("VISA session (for class)"=w10, "error in (no error)"=w9) -> ("VISA session"=w8:refnum<visa-resource-name>, "error out"=w7:errorcluster)  [unwired: 16 in]
  n158 = call "SR7230 Close.vi"("error in (no error)"=w7, "VISA session"=w8) -> ("error out"=w6:errorcluster)
  n159 = call "Error_handler.vi"("error constant"=w6) -> ()
